vi "autocalculate.vi"() -> ()   [LabVIEW 2019]
panel:
  out "output":dbl
  in  "input":dbl
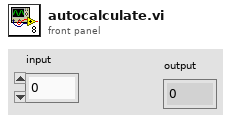
[diagram p1: front panel]
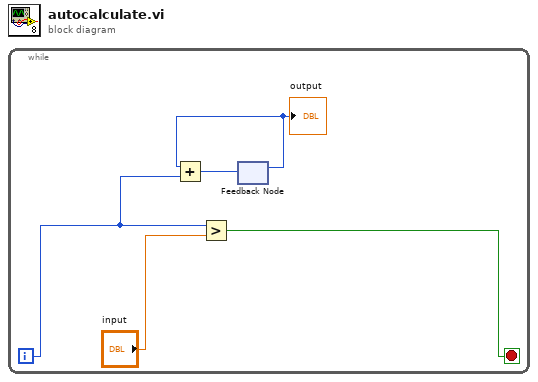
[diagram p0: block diagram]
diagram:
  n1 = while {
    i -> [w3]
    stop <- w4 stop-if-true
    n2 = Greater?(x=w3, y="input") -> (0:w4:bool)
    n3 = feedback #1() -> (w1:i32)  [unwired: 1 in]
    "output" <- w1
    n4 = Add(x=w1, y=w3) -> (x+y=w2:i32)
    n5 = feedback-in #1(w2) -> ()
  }
